vi "increment.vi"(0 "HB_PollingAgent in":refnum<class "HB_PollingAgent.lvclass">, 7 "T:Yes,F:No":bool, 11 "error in (no error)":errorcluster) -> (4 "HB_PollingAgent out":refnum<class "HB_PollingAgent.lvclass">, 15 "error out":errorcluster)   [LabVIEW 2009, in "HB_PollingAgent.lvlib" / "HB_PollingAgent.lvclass"]
uses:
  HB_PollingAgent.lvclass
  HB_PollingAgent.lvclass/HB_PollingAgent.ctl
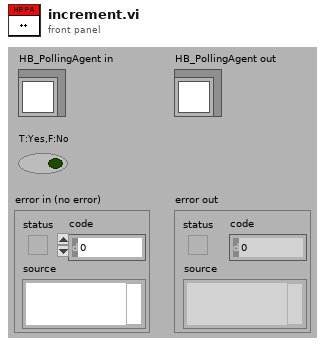
[diagram p1: front panel]
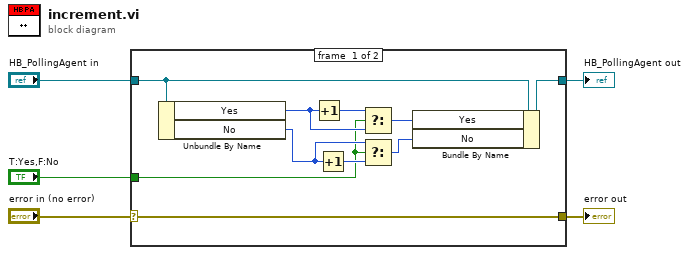
[diagram p0: block diagram]
diagram:
  n1 = case shown="No Error" "error in (no error)" {
    selector: "error in (no error)" -> [w15 w17]
    tunnel: [w15 w17] -> w4
    tunnel: [w13 w16] -> w2
    tunnel: "HB_PollingAgent in" -> [w14 w16]
    tunnel: "T:Yes,F:No" -> [w8 _]
    frame #0 {
      n2 = Unbundle By Name(w14) -> ("Yes"=w11:u32, "No"=w9:u32)
      n3 = Increment(x=w11) -> (x+1=w12:u32)
      n4 = Increment(x=w9) -> (x+1=w10:u32)
      n5 = Select(t=w12, s=w8, f=w11) -> (s? t:f=w7:u32)
      n6 = Select(t=w9, s=w8, f=w10) -> (s? t:f=w6:u32)
      n7 = Bundle By Name(cluster=w14, "Yes"=w7, "No"=w6) -> (w13:refnum<class "HB_PollingAgent.lvclass">)
    }
    frame #1 {
    }
  }
  "error out" <- w4
  "HB_PollingAgent out" <- w2
